vi "Color to HSV.vi"(11 "Color Box":u32(colorbox)) -> (1 "Value (0-255)":u8, 2 "Saturation (0-255)":u8=1, 3 "Hue (0-180)":u8)   [LabVIEW 2014, in "QwaveSys Raspberry Pi Library.lvlib"]
uses:
  QwaveSys Raspberry Pi Library.lvlib
panel:
  out "B":u8
  out "G":u8
  out "R":u8
  out "Color Box Out":u32(colorbox)
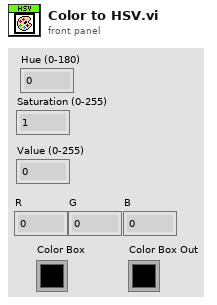
[diagram p1: front panel]
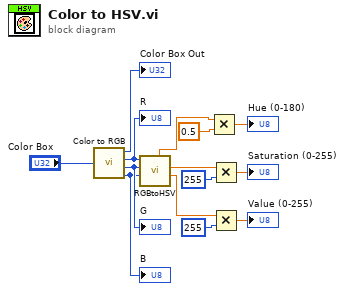
[diagram p0: block diagram]
diagram:
  n1 = call <vilib>:"Color to RGB.vi"("Color"="Color Box") -> ("Resolved Color"=→"Color Box Out":u32, "R"=w12:u8, "G"=w11:u8, "B"=w10:u8)
  "R" <- w12
  "G" <- w11
  "B" <- w10
  n2 = call "RGBtoHSV.vi"("Blue"=w10, "Green"=w11, "Red"=w12) -> ("Value"=w3:dbl, "Saturation"=w5:dbl, "Hue (0-360)"=w9:dbl)  [unwired: 5 in, 1 out]
  n3 = Multiply(x=w9, y=0.5) -> (x*y=→"Hue (0-180)":dbl)
  n4 = Multiply(x=w5, y=u8 255) -> (x*y=→"Saturation (0-255)":dbl)
  n5 = Multiply(x=w3, y=u8 255) -> (x*y=→"Value (0-255)":dbl)
